vi "Route Start Trigger.vi"(6 "trigger master index":i32, 8 "error in":errorcluster, 10 "start trigger rtsi line":string, 11 "fpga interfaces in":refnum<k20>[](array[refnum])) -> (0 "error out":errorcluster, 3 "fpga interfaces out":refnum<k20>[](array[refnum]))   [LabVIEW 2019, in "GettingStarted_5775_Host.lvlib"]
uses:
  GettingStarted_5775_Host.lvlib
  <instrlib>/FlexRIO/API/Host/v1/NI FlexRIO/API/Configure Digital Edge Start Trigger.vi
  <instrlib>/FlexRIO/API/Host/v1/NI FlexRIO/API/Get Property Reference - Fpga Small.vi
  <instrlib>/FlexRIO/API/Host/v1/NI FlexRIO API v1.lvlib
  <resource>/objmgr/sessionReference.rc
  <resource>/objmgr/niflexrioapi.rc
  <resource>/objmgr/niflexrioapiTrigger.rc
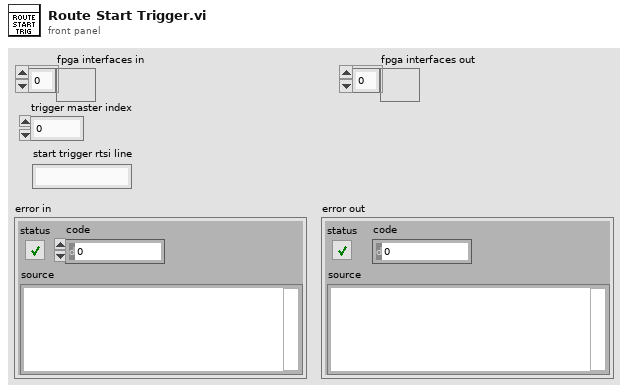
[diagram p1: front panel]
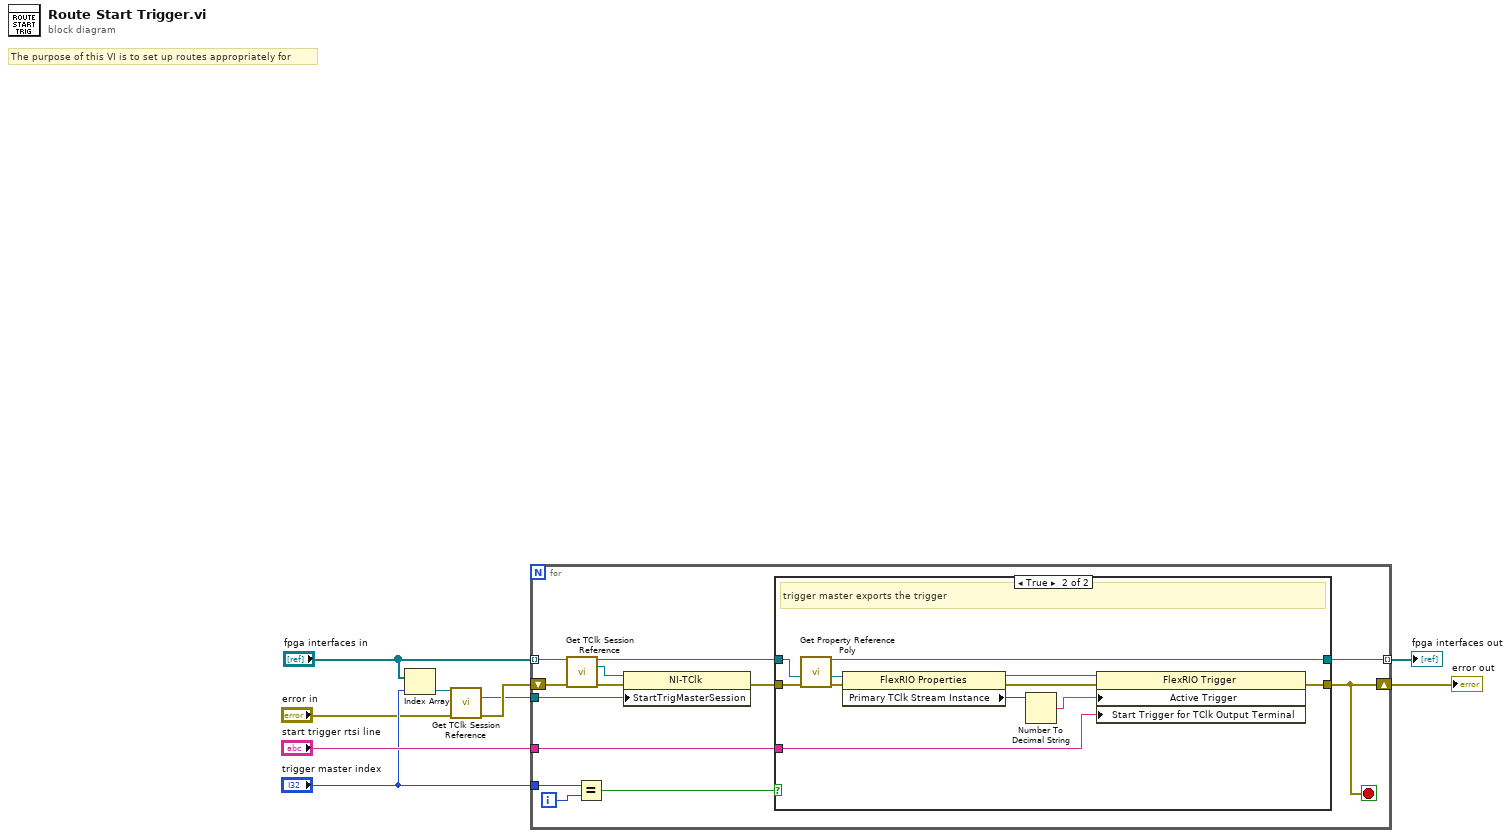
[diagram p0: block diagram]
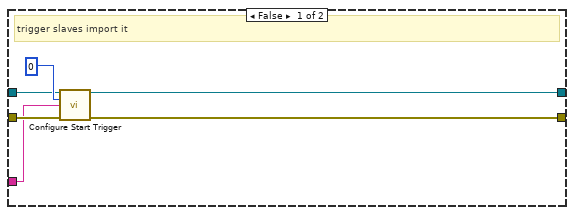
[diagram p2: hidden frame]
diagram:
  # "The purpose of this VI is to set up routes appropriately for"
  n1 = Index Array(array="fpga interfaces in", index="trigger master index") -> (element=w3:refnum<k20>)
  n2 = call <instrlib>:"Get TClk Session Reference.vi"("fpga interface in"=w3, "error in"="error in") -> ("tclk session reference"=w2:refnum<k20>, "error out"=w4:errorcluster)  [unwired: 11 in, 1 out]
  n3 = for {
    tunnel: "start trigger rtsi line" -> [w12]
    shift-right: [w10] -> w8
    shift-left: w4 -> [w19]
    tunnel: "trigger master index" -> [w21]
    tunnel: "fpga interfaces in" -> [w20] mode=indexing
    tunnel: w2 -> [w18]
    tunnel: [w11] -> w1 mode=indexing
    i -> [w22]
    stop <- w10 stop-if-true
    n4 = call <instrlib>:"Get TClk Session Reference.vi"("fpga interface in"=w20, "error in"=w19) -> ("fpga interface out"=w13:refnum<k20>, "tclk session reference"=w16:refnum<k20>, "error out"=w17:errorcluster)  [unwired: 11 in]
    n5 = Equal?(x=w21, y=w22) -> (x = y?=w15:bool)
    n6 = property class="NI-TClk"(reference=w16, error in=w17, "StartTrigMasterSession"=w18) -> (error out=w14:errorcluster)  [unwired: 1 out]
    n7 = case shown="True" w15 {
      tunnel: w14 -> [w28 w36]
      tunnel: w13 -> [w26 w37]
      tunnel: w12 -> [w25 w34]
      tunnel: [w24 w29] -> w11
      tunnel: [w23 w30] -> w10
      frame False {
        # "trigger slaves import it"
        n8 = call-poly <instrlib>:"Configure Start Trigger.vi"("fpga interface in"=w26, "trigger instance"=u32 0, "trigger source"=w25, "error in"=w28) -> ("fpga interface out"=w24:refnum<k20>, "error out"=w23:errorcluster)  [unwired: 9 in, 1 out]
      }
      frame True {
        # "trigger master exports the trigger"
        n9 = call-poly <instrlib>:"Get Property Reference Poly.vi"("error in (no error)"=w36, "fpga interface in"=w37) -> ("error out"=w38:errorcluster, "property reference"=w39:refnum<k20>, "fpga interface out"=w29:refnum<k20>)  [unwired: 4 in]
        n10 = property class="FlexRIO Properties"(reference=w39, error in=w38) -> (reference out=w33:refnum<k20>, error out=w35:errorcluster, "Primary TClk Stream Instance"=w32:i32)
        n11 = Number To Decimal String(number=w32) -> (decimal integer string=w31:string)  [unwired: 1 in]
        n12 = property class="FlexRIO Trigger"(reference=w33, error in=w35, "Active Trigger"=w31, "Start Trigger for TClk Output Terminal"=w34) -> (error out=w30:errorcluster)  [unwired: 1 out]
      }
    }
  }
  "error out" <- w8
  "fpga interfaces out" <- w1
